vi "Slalom Path.vi"   [LabVIEW 2019]
uses:
  Robot Global Data.vi
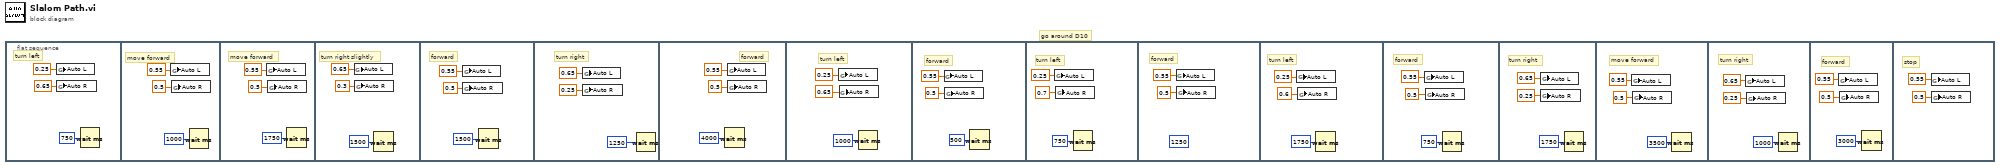
[diagram p0: block diagram]
diagram:
  # "go around D10"
  n1 = flat-sequence {
    frame #0 {
      # "turn left"
      n2 = global write "Robot Global Data.vi" "Auto L"(0.25 ("Auto L")) -> ()
      n3 = global write "Robot Global Data.vi" "Auto R"(0.65 ("Auto R")) -> ()
      n4 = Wait (ms)(milliseconds to wait=u32 750) -> ()  [unwired: 1 out]
    }
    frame #1 {
      # "move forward"
      n5 = global write "Robot Global Data.vi" "Auto L"(0.55 ("Auto L")) -> ()
      n6 = global write "Robot Global Data.vi" "Auto R"(0.5 ("Auto R")) -> ()
      n7 = Wait (ms)(milliseconds to wait=u32 1000) -> ()  [unwired: 1 out]
    }
    frame #2 {
      # "move forward"
      n8 = global write "Robot Global Data.vi" "Auto L"(0.55 ("Auto L")) -> ()
      n9 = global write "Robot Global Data.vi" "Auto R"(0.5 ("Auto R")) -> ()
      n10 = Wait (ms)(milliseconds to wait=u32 1750) -> ()  [unwired: 1 out]
    }
    frame #3 {
      # "turn right slightly"
      n11 = global write "Robot Global Data.vi" "Auto L"(0.65 ("Auto L")) -> ()
      n12 = global write "Robot Global Data.vi" "Auto R"(0.3 ("Auto R")) -> ()
      n13 = Wait (ms)(milliseconds to wait=u32 1500) -> ()  [unwired: 1 out]
    }
    frame #4 {
      # "forward"
      n14 = global write "Robot Global Data.vi" "Auto L"(0.55 ("Auto L")) -> ()
      n15 = global write "Robot Global Data.vi" "Auto R"(0.5 ("Auto R")) -> ()
      n16 = Wait (ms)(milliseconds to wait=u32 1500) -> ()  [unwired: 1 out]
    }
    frame #5 {
      # "turn right"
      n17 = global write "Robot Global Data.vi" "Auto L"(0.65 ("Auto L")) -> ()
      n18 = global write "Robot Global Data.vi" "Auto R"(0.25 ("Auto R")) -> ()
      n19 = Wait (ms)(milliseconds to wait=u32 1250) -> ()  [unwired: 1 out]
    }
    frame #6 {
      # "forward"
      n20 = Wait (ms)(milliseconds to wait=u32 4000) -> ()  [unwired: 1 out]
      n21 = global write "Robot Global Data.vi" "Auto L"(0.55 ("Auto L")) -> ()
      n22 = global write "Robot Global Data.vi" "Auto R"(0.5 ("Auto R")) -> ()
    }
    frame #7 {
      # "turn left"
      n23 = global write "Robot Global Data.vi" "Auto L"(0.25 ("Auto L")) -> ()
      n24 = global write "Robot Global Data.vi" "Auto R"(0.65 ("Auto R")) -> ()
      n25 = Wait (ms)(milliseconds to wait=u32 1000) -> ()  [unwired: 1 out]
    }
    frame #8 {
      # "forward"
      n26 = global write "Robot Global Data.vi" "Auto L"(0.55 ("Auto L")) -> ()
      n27 = global write "Robot Global Data.vi" "Auto R"(0.5 ("Auto R")) -> ()
      n28 = Wait (ms)(milliseconds to wait=u32 500) -> ()  [unwired: 1 out]
    }
    frame #9 {
      # "turn left"
      n29 = global write "Robot Global Data.vi" "Auto L"(0.25 ("Auto L")) -> ()
      n30 = global write "Robot Global Data.vi" "Auto R"(0.7 ("Auto R")) -> ()
      n31 = Wait (ms)(milliseconds to wait=u32 750) -> ()  [unwired: 1 out]
    }
    frame #10 {
      (unwired) u32 1250 ("milliseconds to wait")
      # "forward"
      n32 = global write "Robot Global Data.vi" "Auto L"(0.55 ("Auto L")) -> ()
      n33 = global write "Robot Global Data.vi" "Auto R"(0.5 ("Auto R")) -> ()
    }
    frame #11 {
      # "turn left"
      n34 = global write "Robot Global Data.vi" "Auto L"(0.25 ("Auto L")) -> ()
      n35 = global write "Robot Global Data.vi" "Auto R"(0.6 ("Auto R")) -> ()
      n36 = Wait (ms)(milliseconds to wait=u32 1750) -> ()  [unwired: 1 out]
    }
    frame #12 {
      # "forward"
      n37 = global write "Robot Global Data.vi" "Auto L"(0.55 ("Auto L")) -> ()
      n38 = global write "Robot Global Data.vi" "Auto R"(0.5 ("Auto R")) -> ()
      n39 = Wait (ms)(milliseconds to wait=u32 750) -> ()  [unwired: 1 out]
    }
    frame #13 {
      # "turn right"
      n40 = global write "Robot Global Data.vi" "Auto L"(0.65 ("Auto L")) -> ()
      n41 = global write "Robot Global Data.vi" "Auto R"(0.25 ("Auto R")) -> ()
      n42 = Wait (ms)(milliseconds to wait=u32 1750) -> ()  [unwired: 1 out]
    }
    frame #14 {
      # "move forward"
      n43 = global write "Robot Global Data.vi" "Auto L"(0.55 ("Auto L")) -> ()
      n44 = global write "Robot Global Data.vi" "Auto R"(0.5 ("Auto R")) -> ()
      n45 = Wait (ms)(milliseconds to wait=u32 3500) -> ()  [unwired: 1 out]
    }
    frame #15 {
      # "turn right"
      n46 = global write "Robot Global Data.vi" "Auto L"(0.65 ("Auto L")) -> ()
      n47 = global write "Robot Global Data.vi" "Auto R"(0.25 ("Auto R")) -> ()
      n48 = Wait (ms)(milliseconds to wait=u32 1000) -> ()  [unwired: 1 out]
    }
    frame #16 {
      # "forward"
      n49 = global write "Robot Global Data.vi" "Auto L"(0.55 ("Auto L")) -> ()
      n50 = global write "Robot Global Data.vi" "Auto R"(0.5 ("Auto R")) -> ()
      n51 = Wait (ms)(milliseconds to wait=u32 3000) -> ()  [unwired: 1 out]
    }
    frame #17 {
      # "stop"
      n52 = global write "Robot Global Data.vi" "Auto L"(0.55 ("Auto L")) -> ()
      n53 = global write "Robot Global Data.vi" "Auto R"(0.5 ("Auto R")) -> ()
    }
  }
